vi "VII Scan Device.vi"(11 "NeedInit":u8) -> (3 "function return":i32)   [LabVIEW 2010, in "ControlI2C.lvlib"]
doc: "int __stdcall VII_ScanDevice(unsigned char NeedInit=1);"
uses:
  ControlI2C.lvlib
  ControlI2C/Ginkgo_Driver.dll
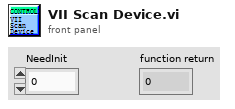
[diagram p1: front panel]
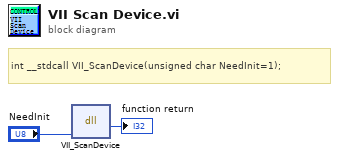
[diagram p0: block diagram]
diagram:
  # "int __stdcall VII_ScanDevice(unsigned char NeedInit=1);"
  n1 = dll-call lib="E:/Project/vt_ginkgo/truck/Ginkgo Driver/vs2010/Ginkgo_USB-I2C&SPI&CAN_API_v2.0.3.3/lib/labview_32bit/ControlI2C/Ginkgo_Driver.*" fn="VII_ScanDevice"("NeedInit"="NeedInit") -> (→"function return":i32)  [unwired: 4 in, 2 out]
